vi "DBClient1.vi"() -> ()   [LabVIEW 2015]
uses:
  <vilib>/addons/database/Connection.llb/DB Tools Open Connec (Path).vi
  <vilib>/addons/database/Connection.llb/Conn Execute.vi
  <vilib>/addons/database/Recordset.llb/Rec Fetch Recordset Data (R).vi
  <vilib>/addons/database/Recordset.llb/Rec Destroy - Connection.vi
  <vilib>/addons/database/_DB Variant To Data/Database Variant To Data.xnode
  <vilib>/addons/database/NI_Database_API.lvlib
panel:
  in  "stop":bool
  out "Tabel Buku":string[][](table)
  in  "Search Button":bool
  in  "Search":string
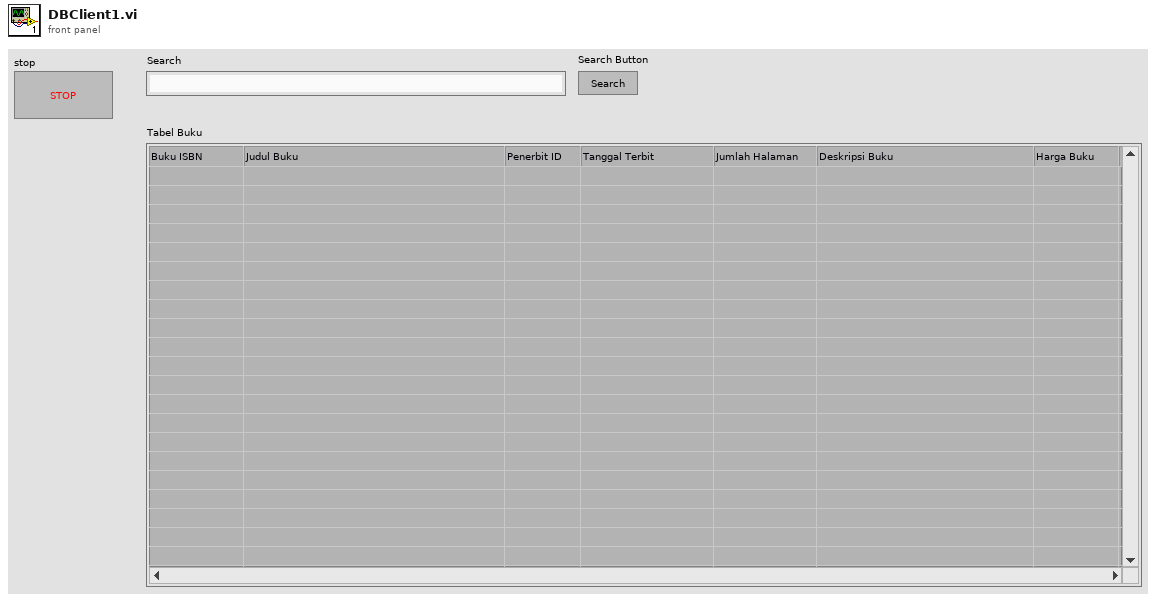
[diagram p1: front panel]
types:
  T1 = typedef "NI_Database_API.lvlib/Conn ObjectReference.ctl" = refnum<k1>
  T2 = typedef "NI_Database_API.lvlib/Rec ObjectReference.ctl" = refnum<k1>
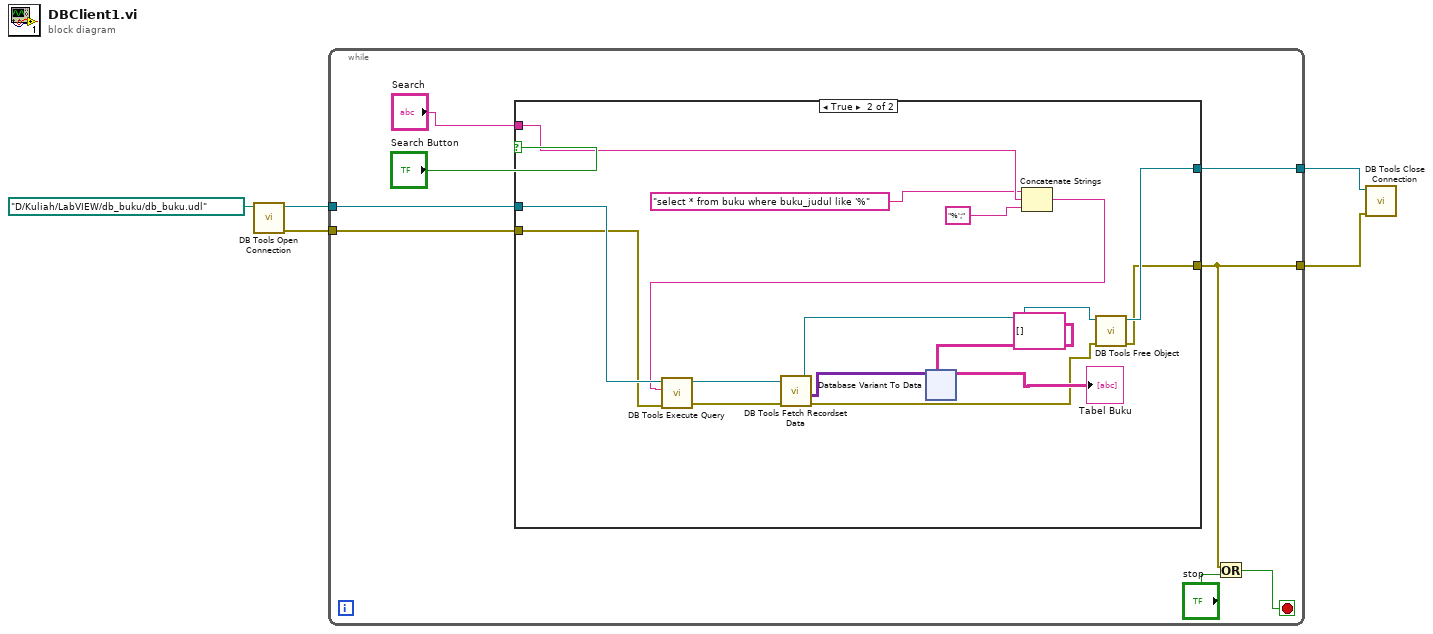
[diagram p0: block diagram]
diagram:
  n1 = call-poly <vilib>:"DB Tools Open Connection.vi"("connection information"=path "D:/Kuliah/LabVIEW/db_buku/db_buku.udl") -> ("error out"=w4:errorcluster, "connection reference"=w5:T1)  [unwired: 7 in]
  n2 = while {
    tunnel: w5 -> [w11]
    tunnel: w4 -> [w10]
    tunnel: [w9] -> w3
    tunnel: [w8] -> w2
    stop <- w6 stop-if-true
    n3 = case shown="True" "Search Button" {
      tunnel: "Search" -> [_ w19]
      tunnel: w11 -> [w15 w25]
      tunnel: w10 -> [w14 w24]
      tunnel: [w15 w21] -> w9
      tunnel: [w14 w20] -> w8
      frame False {
      }
      frame True {
        n4 = Concatenate Strings("select * from buku where buku_judul like '%" ("string"), w19, "%';" ("string")) -> (w18:string)
        n5 = call-poly <vilib>:"DB Tools Execute Query.vi"("error in (no error)"=w24, "SQL query"=w18, "connection reference"=w25) -> ("error out"=w29:errorcluster, "recordset reference"=w30:T2)  [unwired: 5 in]
        n6 = call-poly <vilib>:"DB Tools Fetch Recordset Data.vi"("error in (no error)"=w29, "recordset reference"=w30) -> ("error out"=w23:errorcluster, "recordset data"=w28:variant[][], "recordset reference out"=w22:T2)  [unwired: 3 in]
        n7 = xnode "Database Variant To Data"("database variant"=w28, "type"=string[][] []) -> ("data"=→"Tabel Buku":string[][])  [unwired: 1 in, 1 out]
        n8 = call-poly <vilib>:"DB Tools Free Object.vi"("error in (no error)"=w23, "recordset reference"=w22) -> ("error out"=w20:errorcluster, "connection reference"=w21:T1)  [unwired: 8 in]
      }
    }
    n9 = Or(x=w8, y="stop") -> (x .or. y?=w6:bool)
  }
  n10 = call <vilib>:"DB Tools Close Connection.vi"("error in (no error)"=w2, "connection reference"=w3) -> ()  [unwired: 5 in, 1 out]
